vi "FGV_DOCK_config_info.vi"(7 "options":T4=enum."get", 8 "error_in":errorcluster, 10 "input":variant, 11 "all_config_info_in":T1={"main_ini_file"={"SQL Driver"="", "SQL Server"="", "SQL Database"="", "SQL UID"="", "Reference table"="", "Reference history"="", "Archivisation CFG table"="", "Archivisation CFG history"="", "User table"="", "User history"="", "default language"="", "SCANNER COM port"=0, "SCANNER Baud rate"=0, "SCANNER Data bits"=0, "SCANNER Pairity"=enum."None", "SCANNER Stop bits"=10, "SCANNER Flow control"=0, "SCANNER Termination char"=0, "PRINTER PC port"=0, "PRINTER IP"="", "PRINTER port"=0, "PRINTER Keep alive timer [ms]"=0, "logout timeout [ms]"=0}, "SQL Password"="", "PRINTER Label"="", "PRINTER Template"="", "Last Label"="", "queue_refnums"={"MAIN_queue"=refnum, "SCANNER_queue"=refnum, "SCANNER_login"=refnum, "PRINTER_queue"=refnum}} {"main_ini_file"."SCANNER Flow control" items=["None"=0, "XON/XOFF"=1, "RTS/CTS"=2, "DTR/DSR"=4]; "main_ini_file"."SCANNER Stop bits" items=["1.0"=10, "1.5"=15, "2.0"=20]}) -> (0 "error_out":errorcluster, 3 "all_config_info_out":T1={"main_ini_file"={"SQL Driver"="", "SQL Server"="", "SQL Database"="", "SQL UID"="", "Reference table"="", "Reference history"="", "Archivisation CFG table"="", "Archivisation CFG history"="", "User table"="", "User history"="", "default language"="", "SCANNER COM port"=0, "SCANNER Baud rate"=0, "SCANNER Data bits"=0, "SCANNER Pairity"=enum."None", "SCANNER Stop bits"=10, "SCANNER Flow control"=0, "SCANNER Termination char"=0, "PRINTER PC port"=0, "PRINTER IP"="", "PRINTER port"=0, "PRINTER Keep alive timer [ms]"=0, "logout timeout [ms]"=0}, "SQL Password"="", "PRINTER Label"="", "PRINTER Template"="", "Last Label"="", "queue_refnums"={"MAIN_queue"=refnum, "SCANNER_queue"=refnum, "SCANNER_login"=refnum, "PRINTER_queue"=refnum}} {"main_ini_file"."SCANNER Flow control" items=["None"=0, "XON/XOFF"=1, "RTS/CTS"=2, "DTR/DSR"=4]; "main_ini_file"."SCANNER Stop bits" items=["1.0"=10, "1.5"=15, "2.0"=20]})   [LabVIEW 2019]
uses:
  FGV_DOCK_config_info.ctl
  ini/typedef/DOCK_all_config_info.ctl
  ini/typedef/DOCK_main_ini_file.ctl
  queues/typedef/DOCK_queue_refnums.ctl
  queues/typedef/DOCK_MAIN_queue_element.ctl
  MAIN/DOCK_MAIN_sequence_state.ctl
  queues/typedef/DOCK_SCANNER_queue_element.ctl
  SCANNER/DOCK_SCANNER_sequence_state.ctl
  queues/typedef/DOCK_PRINTER_queue_element.ctl
  PRINTER/DOCK_PRINTER_sequence_state.ctl
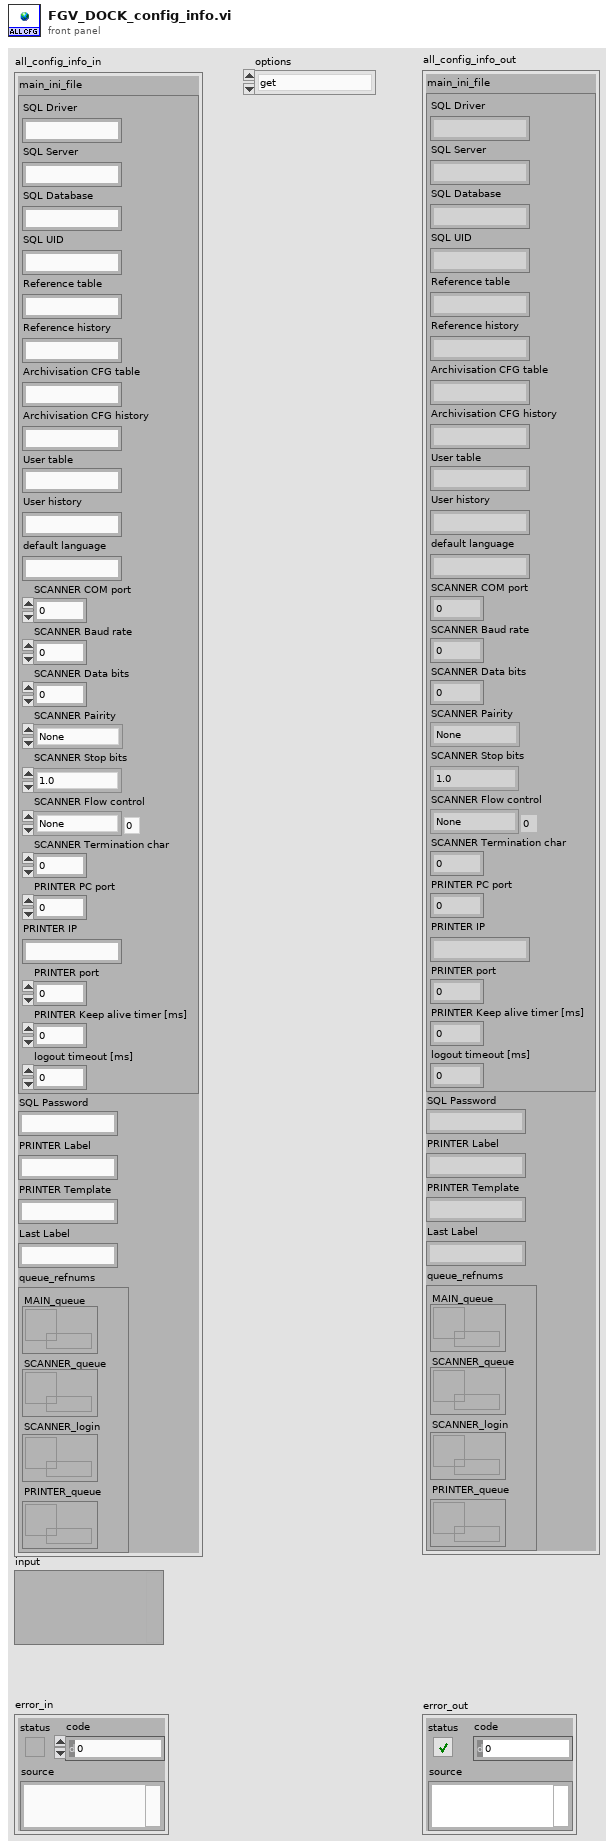
[diagram p1: front panel]
types:
  T1 = typedef "DOCK_all_config_info.ctl" = cluster{"main_ini_file":T2, "SQL Password":string, "PRINTER Label":string, "PRINTER Template":string, "Last Label":string, "queue_refnums":T3}
  T2 = typedef "DOCK_main_ini_file.ctl" = cluster{"SQL Driver":string, "SQL Server":string, "SQL Database":string, "SQL UID":string, "Reference table":string, "Reference history":string, "Archivisation CFG table":string, "Archivisation CFG history":string, "User table":string, "User history":string, "default language":string, "SCANNER COM port":u16, "SCANNER Baud rate":u32, "SCANNER Data bits":u16, "SCANNER Pairity":enum16{"None", "Odd", "Even", "Mark", "Space"}, "SCANNER Stop bits":u16, "SCANNER Flow control":u16, "SCANNER Termination char":u8, "PRINTER PC port":u16, "PRINTER IP":string, "PRINTER port":u16, "PRINTER Keep alive timer [ms]":i32, "logout timeout [ms]":i32}
  T3 = typedef "DOCK_queue_refnums.ctl" = cluster{"MAIN_queue":refnum<queue>, "SCANNER_queue":refnum<queue>, "SCANNER_login":refnum<queue>, "PRINTER_queue":refnum<queue>}
  T4 = typedef "FGV_DOCK_config_info.ctl" = enum16{"initialize", "set", "set_last_label", "get"}
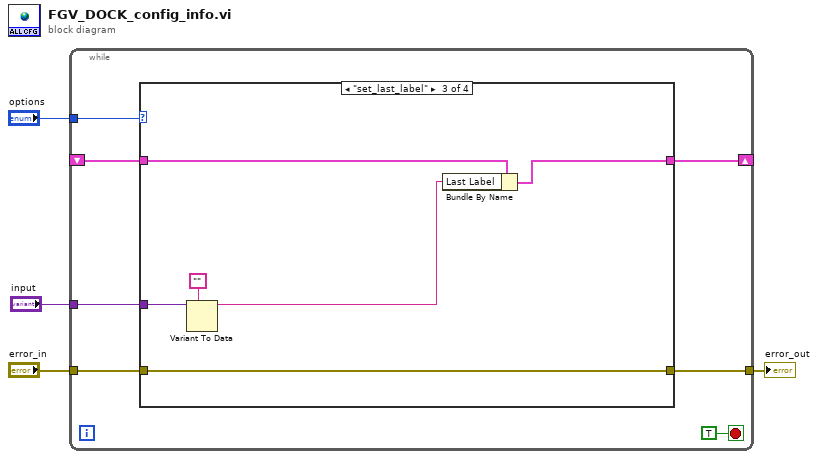
[diagram p0: block diagram]
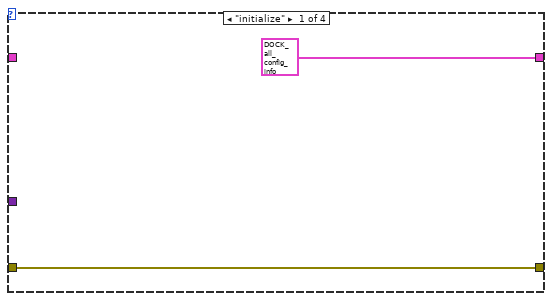
[diagram p2: hidden frame]
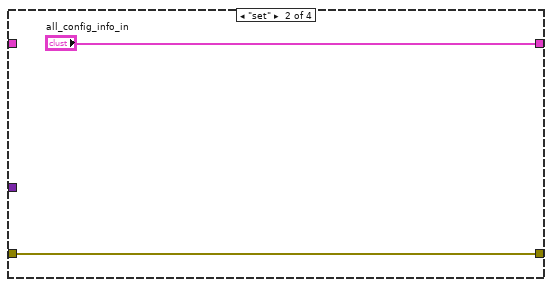
[diagram p3: hidden frame]
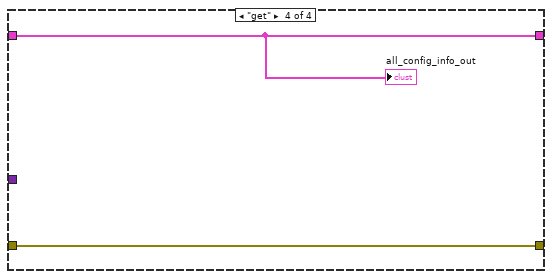
[diagram p4: hidden frame]
diagram:
  n1 = while {
    tunnel: "options" -> [w10]
    tunnel: [w9] -> w3
    tunnel: "error_in" -> [w8]
    shift-right: [w6] -> _
    shift-left: _ -> [w7]
    tunnel: "input" -> [w5]
    stop <- TRUE stop-if-true
    n2 = case shown="\"set_last_label\"" w10 {
      tunnel: [w13 w15 w21 w23] -> w9
      tunnel: w8 -> [w13 w15 w21 w23]
      tunnel: [T1 {"main_ini_file"={"SQL Driver"="", "SQL Server"="", "SQL Database"="", "SQL UID"="", "Reference table"="", "Reference history"="", "Archivisation CFG table"="", "Archivisation CFG history"="", "User table"="", "User history"="", "default language"="", "SCANNER COM port"=0, "SCANNER Baud rate"=0, "SCANNER Data bits"=0, "SCANNER Pairity"=enum."None", "SCANNER Stop bits"=10, "SCANNER Flow control"=0, "SCANNER Termination char"=0, "PRINTER PC port"=0, "PRINTER IP"="", "PRINTER port"=0, "PRINTER Keep alive timer [ms]"=0, "logout timeout [ms]"=0}, "SQL Password"="", "PRINTER Label"="", "PRINTER Template"="", "Last Label"="", "queue_refnums"={"MAIN_queue"=refnum, "SCANNER_queue"=refnum, "SCANNER_login"=refnum, "PRINTER_queue"=refnum}} ("all_config_info_out") "all_config_info_in" w17 w22] -> w6
      tunnel: w7 -> [_ _ w18 w22]
      tunnel: w5 -> [_ _ w20 _]
      frame "initialize" {
      }
      frame "set" {
      }
      frame "set_last_label" {
        n3 = Variant To Data(type="", Variant=w20) -> (data=w16:string)  [unwired: 1 in, 1 out]
        n4 = Bundle By Name(cluster=w18, "Last Label"=w16) -> (w17:T1)
      }
      frame "get" {
        "all_config_info_out" <- w22
      }
    }
  }
  "error_out" <- w3
